vi "Close PDF.vi"(0 "PDF Report":refnum<class "PDF Report Class.lvclass">, 11 "error in (no error)":errorcluster) -> (4 "Path":path, 15 "error out":errorcluster)   [LabVIEW 2020, in "Exaprom PDF.lvlib"]
doc: "Closes the PDF report and, if necessary, appends headers, footers and the watermark.\n\n<B>FRANÇAIS</B>\nCe VI ferme le rapport PDF et, si nécessaire, ajoute les en-tête, pieds de page et filigrane.\n\nVersion 1.1\nDeveloped by Jean-Marc Simard\nCopyright © 2012, Exaprom Inc.\nAll rights reserved.\nLicense: BSD\n\nWith iTextSharp 4.1.6 (http://itextsharp.sourceforge.net)\nunder Mozilla Public License Version 1.1\n(http://www.mozilla.org/MPL/MPL-1.1.html)"
uses:
  <userlib>/labview-PDF-writer-master/Exaprom PDF.lvlib
  <userlib>/labview-PDF-writer-master/LV Class/PDF Report Class/PDF Report Class.lvclass
  C:/Program Files (x86)/National Instruments/LabVIEW 2020/user.lib/labview-PDF-writer-master/DLL/itextsharp.dll
  DLL/itextsharp.dll
  <userlib>/labview-PDF-writer-master/LV Class/Header and Footer Class/Header and Footer Class.lvclass
  <userlib>/labview-PDF-writer-master/LV Class/Fonts Class/Font Class.lvclass
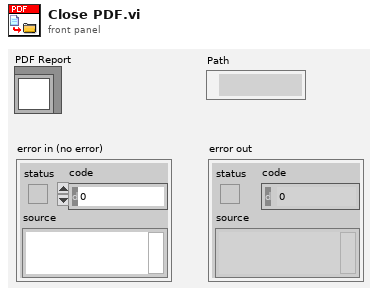
[diagram p1: front panel]
types:
  T1 = typedef "Exaprom PDF.lvlib/PDF File and position.ctl" = cluster{"Path":path, "Pages":string, "Source":T2, "Start at page old":i32, "Start at page new":i32, "Owner password":string}
  T2 = typedef "Exaprom PDF.lvlib/PDF file source.ctl" = enum16{"PDF Report", "File to add"}
  T3 = typedef "Exaprom PDF.lvlib/Header and Footer Class.lvclass/Header Footer cluster V2.ctl" = cluster{"Header or Footer":T4, "Start page":i32, "Start with #":i32, "Type":T5, "Alignment":T6, "Vertical Alignement":T7, "Line spacing":T8, "Image (%)":sgl, "Page #":T9, "Text":string, "Path":string, "Font":T10, "Font refnum":refnum<k24>, "Line":cluster{"Line":T15, "Thickness (points)":sgl, "Colour":T12}, "Vert margin":dbl, "Hyperlink":string}
  T4 = typedef "Exaprom PDF.lvlib/Header or Footer.ctl" = enum16{"Header", "Footer"}
  T5 = typedef "Exaprom PDF.lvlib/Header Footer Type.ctl" = enum16{"Select", "Text", "Text + hyperlink", "Page number", "Image", "Image + hyperlink"}
  T6 = typedef "Exaprom PDF.lvlib/Header footer horiz alignment.ctl" = enum16{"Left", "Center", "Right"}
  T7 = typedef "Exaprom PDF.lvlib/Cell Vertical alignment.ctl" = enum16{"TOP", "MIDDLE", "BOTTOM"}
  T8 = typedef "Exaprom PDF.lvlib/Line spacing.ctl" = enum16{"Select", "1.0", "1.5", "2.0"}
  T9 = typedef "Exaprom PDF.lvlib/Page number.ctl" = cluster{"Text 1":string, "Text 2":string, "Text 3":string}
  T10 = typedef "Exaprom PDF.lvlib/Font complete cluster horizontal.ctl" = cluster{"Name":string, "Size":T11, "Color":T12, "Style":cluster{"Bold":bool, "Italic":bool, "Underline":bool, "Strikeout":bool}, "Type":T13}
  T11 = typedef "Exaprom PDF.lvlib/Font size.ctl" = sgl
  T12 = typedef "Exaprom PDF.lvlib/Font color.ctl" = u32
  T13 = typedef "Exaprom PDF.lvlib/Type and encoding.ctl" = cluster{"Type&direction":T14, "Embedded":bool, "Encoding":string}
  T14 = typedef "Exaprom PDF.lvlib/Type and run direction.ctl" = enum16{"Select", "ASCII", "UTF-16", "UTF-16 (default)", "UTF-16 (LTR)", "UTF-16 (RTL)"}
  T15 = typedef "Exaprom PDF.lvlib/Header Footer Line.ctl" = enum16{"No line", "Horizontal line"}
  T16 = typedef "Exaprom PDF.lvlib/Watermark cluster2.ctl" = cluster{"Show? (F)":bool, "Type":enum16{"Image", "Text"}, "Opacity (%)":sgl, "Rotate(°)":sgl, "Position":cluster{"Position":T17, "X":sgl, "Y":sgl}, "Image path":path, "Scaled(%)":sgl, "Image refnum":refnum<k24>, "Text":string, "Font":cluster{"Name":string, "Size":T11, "Color":T12}, "Font refnum":refnum<k24>, "Alignment":T6, "Automatic":bool}
  T17 = typedef "Exaprom PDF.lvlib/Watermark Position.ctl" = enum16{"Absolute", "Center (page)", "Center (text section)"}
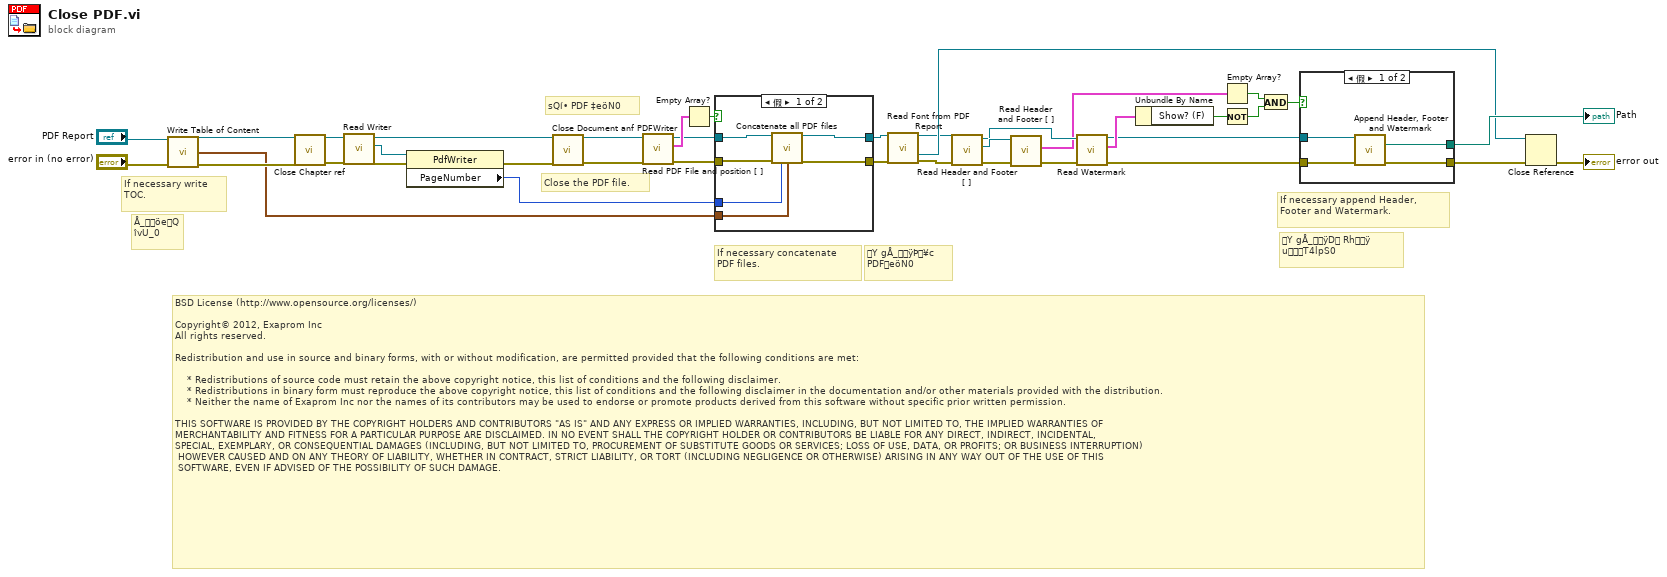
[diagram p0: block diagram]
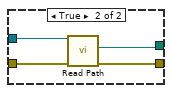
[diagram p3: hidden frame]
diagram:
  # "Y\tgÅ_ÿD Rhÿ\nuT4lpS0"
  # "Y\tgÅ_ÿÞ¥c\nPDFeöN0"
  # "sQí• PDF ‡eöN0"
  # "Å_öeQ\nîvU_0"
  # "If necessary write\nTOC."
  # "If necessary concatenate\nPDF files."
  # "If necessary append Header,\nFooter and Watermark."
  # "Close the PDF file."
  # "BSD License (http://www.opensource.org/licenses/)\n\nCopyright© 2012, Exaprom Inc\nAll rights reserved.\n\nRedistribution and use in source and binary forms, with or without modification, are permitted provided that the following conditions are met:\n\n    * Redistributions of source code must retain the above copyright notice, this list of conditions and the following disclaimer.\n    * Redistributions in binary form must reproduce the above copyright notice, this list of conditions and the following disclaimer in the documentation and/or other materials provided with the distribution.\n    * Neither the name of Exaprom Inc nor the names of its contributors may be used to endorse or promote products derived from this software without specific prior written permission.\n\nTHIS SOFTWARE IS PROVIDED BY THE COPYRIGHT HOLDERS AND CONTRIBUTORS \"AS IS\" AND ANY EXPRESS OR IMPLIED WARRANTIES, INCLUDING, BUT NOT LIMITED TO, THE IMPLIED WARRANTIES OF \nMERCHANTABILITY AND FITNESS FOR A PARTICULAR PURPOSE ARE DISCLAIMED. IN NO EVENT SHALL THE COPYRIGHT HOLDER OR CONTRIBUTORS BE LIABLE FOR ANY DIRECT, INDIRECT, INCIDENTAL,\nSPECIAL, EXEMPLARY, OR CONSEQUENTIAL DAMAGES (INCLUDING, BUT NOT LIMITED TO, PROCUREMENT OF SUBSTITUTE GOODS OR SERVICES; LOSS OF USE, DATA, OR PROFITS; OR BUSINESS INTERRUPTION)\n HOWEVER CAUSED AND ON ANY THEORY OF LIABILITY, WHETHER IN CONTRACT, STRICT LIABILITY, OR TORT (INCLUDING NEGLIGENCE OR OTHERWISE) ARISING IN ANY WAY OUT OF THE USE OF THIS\n SOFTWARE, EVEN IF ADVISED OF THE POSSIBILITY OF SUCH DAMAGE."
  n1 = call <userlib>:"Write Table of Content.vi"("PDF Report IN"="PDF Report", "error in (no error)"="error in (no error)") -> ("PDF Report OUT"=w5:refnum<class "PDF Report Class.lvclass">, "TOC page"=w1:cluster{"Start":i32, "Number":i32}, "error out"=w3:errorcluster)  [unwired: 11 in]
  n2 = call <userlib>:"Close Chapter ref.vi"("PDF Report IN"=w5, "error in (no error)"=w3) -> ("PDF Report OUT"=w4:refnum<class "PDF Report Class.lvclass">, "error out"=w2:errorcluster)  [unwired: 12 in]
  n3 = call-dynamic "Read Writer.vi"("error in (no error)"=w2, "PDF Report Class in"=w4) -> ("error out"=w11:errorcluster, "Writer"=w8:refnum<k24>, "PDF Report Class out"=w12:refnum<class "PDF Report Class.lvclass">)  [unwired: 7 in]
  n4 = property class="PdfWriter"(reference=w8, error in=w11) -> (error out=w10:errorcluster, "PageNumber"=w9:i32)  [unwired: 1 out]
  n5 = call <userlib>:"Close Document anf PDFWriter.vi"("PDF Report IN"=w12, "error in (no error)"=w10) -> ("PDF Report OUT"=w35:refnum<class "PDF Report Class.lvclass">, "error out"=w17:errorcluster)  [unwired: 12 in]
  n6 = call-dynamic "Read PDF File and position [ ].vi"("error in (no error)"=w17, "PDF Report Class in"=w35) -> ("error out"=w16:errorcluster, "PDF File and position [ ]"=w19:T1[], "PDF Report Class out"=w13:refnum<class "PDF Report Class.lvclass">)  [unwired: 7 in]
  n7 = Empty Array?(array=w19) -> (empty?=w18:bool)
  n8 = case shown="假" w18 {
    tunnel: w16 -> [w41 w45]
    tunnel: [w42 w45] -> w15
    tunnel: [w43 w46] -> w14
    tunnel: w13 -> [w44 w46]
    tunnel: w9 -> [w39 _]
    tunnel: w1 -> [w40 _]
    frame False {
      n9 = call <userlib>:"Concatenate all PDF files.vi"("PDF Report IN"=w44, "error in (no error)"=w41, "Last PageNumber"=w39, "TOC page"=w40) -> ("PDF Report OUT"=w43:refnum<class "PDF Report Class.lvclass">, "error out"=w42:errorcluster)  [unwired: 10 in]
    }
    frame True {
    }
  }
  n10 = call <userlib>:"Read Font from PDF Report.vi"("PDF Report"=w14, "error in (no error)"=w15) -> ("PDF Report duplicate"=w26:refnum<class "PDF Report Class.lvclass">, "Font Ref"=w34:refnum<k24>, "error out"=w28:errorcluster)  [unwired: 7 in, 4 out]
  n11 = call-dynamic "Read Header and Footer [ ].vi"("error in (no error)"=w28, "PDF Report Class in"=w26) -> ("error out"=w27:errorcluster, "Header and Footer Class.lvclass"=w25:refnum<class "Header and Footer Class.lvclass">, "PDF Report Class out"=w24:refnum<class "PDF Report Class.lvclass">)  [unwired: 7 in]
  n12 = call-dynamic "Read Header and Footer [ ].vi"("error in (no error)"=w27, "Header and Footer Class in"=w25) -> ("error out"=w23:errorcluster, "Header and Footer [ ]"=w22:T3[])  [unwired: 7 in, 1 out]
  n13 = call-dynamic "Read Watermark .vi"("error in (no error)"=w23, "PDF Report Class in"=w24) -> ("error out"=w33:errorcluster, "Watermark Cluster"=w32:T16, "PDF Report Class out"=w30:refnum<class "PDF Report Class.lvclass">)  [unwired: 7 in]
  n14 = Unbundle By Name(w32) -> ("Show? (F)"=w31:bool)
  n15 = Empty Array?(array=w22) -> (empty?=w21:bool)
  n16 = Not(x=w31) -> (.not. x?=w20:bool)
  n17 = And(x=w21, y=w20) -> (x .and. y?=w37:bool)
  n18 = case shown="假" w37 {
    tunnel: [w50 w51] -> w38
    tunnel: [w49 w53] -> w36
    tunnel: w33 -> [w48 w54]
    tunnel: w30 -> [w47 w52]
    frame False {
      n19 = call <userlib>:"Append Header, Footer and Watermark.vi"("PDF Report IN"=w47, "error in (no error)"=w48) -> ("Path"=w50:path, "error out"=w49:errorcluster)  [unwired: 12 out]
    }
    frame True {
      n20 = call-dynamic "Read Path.vi"("error in (no error)"=w54, "PDF Report Class in"=w52) -> ("error out"=w53:errorcluster, "Path"=w51:path)  [unwired: 7 in, 1 out]
    }
  }
  "Path" <- w38
  n21 = Close Reference(reference=w34, error in (no error)=w36) -> (error out=→"error out":errorcluster)
